vi "Set Database API.vi"(8 "error in (no error)":errorcluster, 10 "Database":refnum<class "Database.lvclass">, 11 "ScriptDialog in":refnum<class "ScriptDialog.lvclass">) -> (0 "error out":errorcluster, 3 "ScriptDialog out":refnum<class "ScriptDialog.lvclass">)   [LabVIEW 2015, in "ScriptDialog.lvclass"]
uses:
  ScriptDialog.lvclass
  _Database/Database.lvclass
  ScriptDialog.lvclass/ScriptDialog.ctl
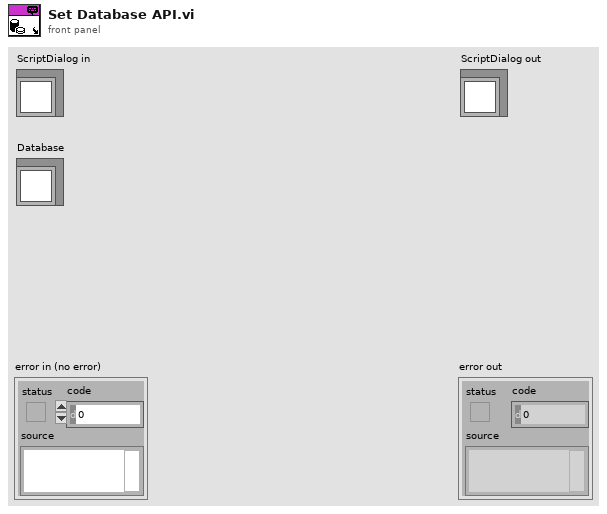
[diagram p1: front panel]
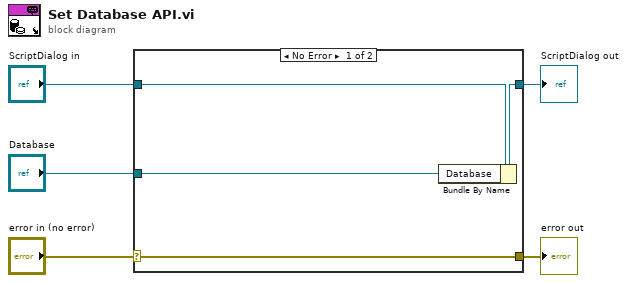
[diagram p0: block diagram]
diagram:
  n1 = case shown="No Error" "error in (no error)" {
    selector: "error in (no error)" -> [w9 w10]
    tunnel: [w9 w10] -> w4
    tunnel: [w7 w11] -> w2
    tunnel: "ScriptDialog in" -> [w8 w11]
    tunnel: "Database" -> [w6 _]
    frame No Error {
      n2 = Bundle By Name(cluster=w8, "Database"=w6) -> (w7:refnum<class "ScriptDialog.lvclass">)
    }
    frame Error {
    }
  }
  "error out" <- w4
  "ScriptDialog out" <- w2
